vi "Status Bar.vi"(0 "Status Bar":refnum<vi>, 5 "Status":string, 11 "error in (no error)":errorcluster, 13 "Operation":T1) -> (15 "error out":errorcluster)   [LabVIEW 2014, in "SLL Application.lvlib"]
uses:
  SLL Application.lvlib
  _Typedefs/Status Bar Operation.ctl
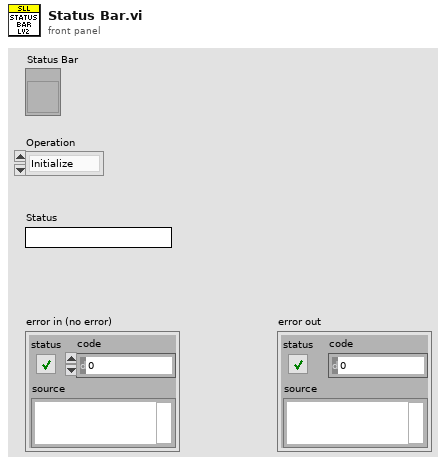
[diagram p1: front panel]
types:
  T1 = typedef "SLL Application.lvlib/Status Bar Operation.ctl" = enum16{"Initialize", "Update", "Clear", "Close"}
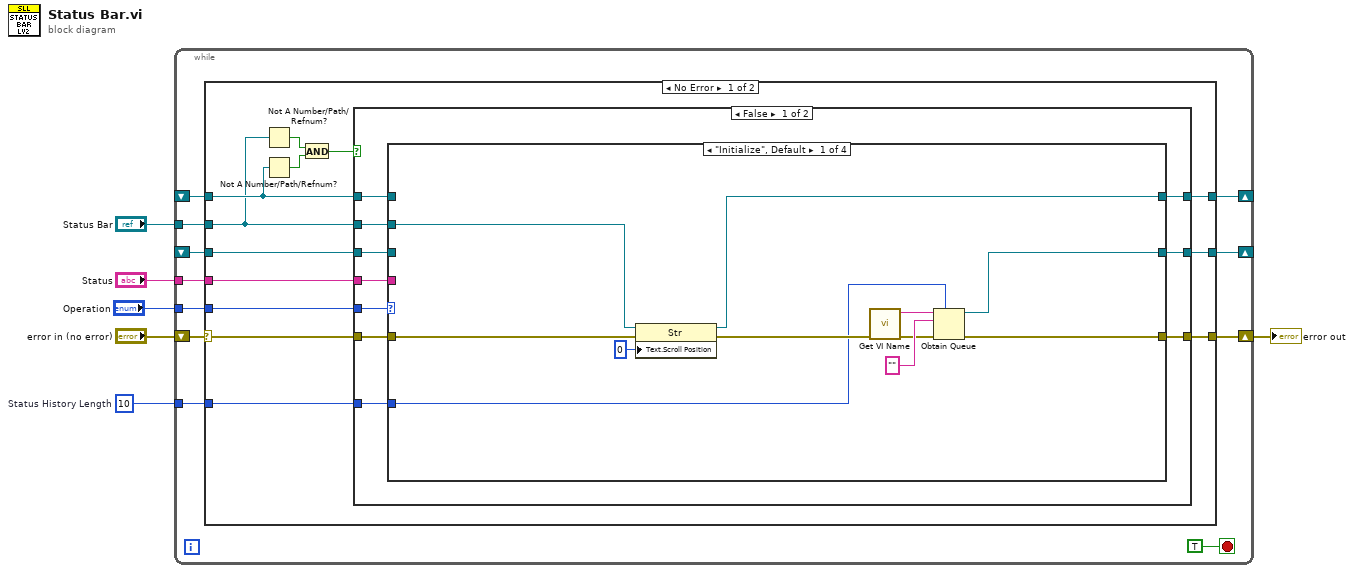
[diagram p0: block diagram]
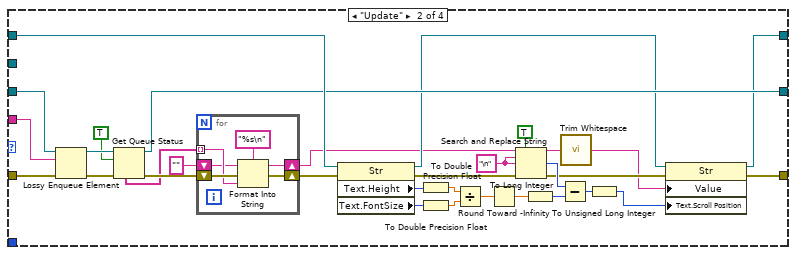
[diagram p2: hidden frame]
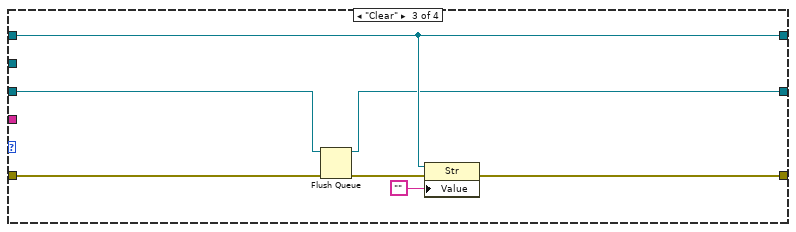
[diagram p3: hidden frame]
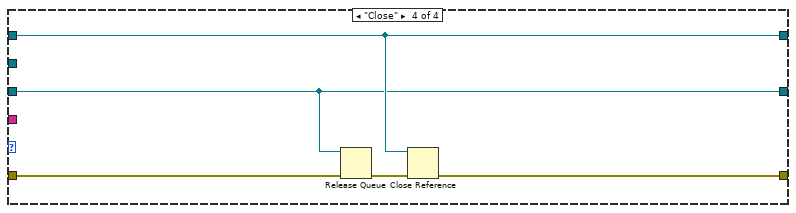
[diagram p4: hidden frame]
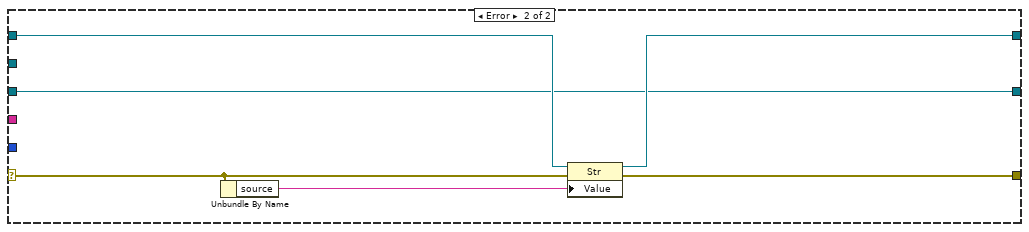
[diagram p6: hidden frame]
diagram:
  w1 = 10  # Status History Length
  n1 = while {
    shift-right: [w16] -> _
    shift-left: _ -> [w17]
    tunnel: "Operation" -> [w15]
    tunnel: "Status Bar" -> [w14]
    shift-right: [w12] -> w4
    shift-left: "error in (no error)" -> [w13]
    tunnel: "Status" -> [w10]
    shift-right: [w9] -> _
    shift-left: _ -> [w8]
    tunnel: w1 -> [w7]
    stop <- TRUE stop-if-true
    n2 = case shown="No Error" w13 {
      selector: w13 -> [w28 w107]
      tunnel: w17 -> [w20 w109]
      tunnel: [w30 w108] -> w16
      tunnel: w15 -> [w29 _]
      tunnel: w14 -> [w19 _]
      tunnel: [w27 w110] -> w12
      tunnel: w10 -> [w26 _]
      tunnel: [w25 w105] -> w9
      tunnel: w8 -> [w24 w105]
      tunnel: w7 -> [w18 _]
      frame No Error {
        n3 = Not A Number/Path/Refnum?(number/path/refnum=w19) -> (NaN/Path/Refnum?=w23:bool)
        n4 = Not A Number/Path/Refnum?(number/path/refnum=w20) -> (NaN/Path/Refnum?=w22:bool)
        n5 = And(x=w23, y=w22) -> (x .and. y?=w21:bool)
        n6 = case shown="False" w21 {
          tunnel: w20 -> [w40 w104]
          tunnel: [w39 w104] -> w30
          tunnel: w29 -> [w38 _]
          tunnel: w19 -> [w37 _]
          tunnel: w28 -> [w36 w102]
          tunnel: [w35 w102] -> w27
          tunnel: w26 -> [w34 _]
          tunnel: [w33 w103] -> w25
          tunnel: w24 -> [w32 w103]
          tunnel: w18 -> [w31 _]
          frame False {
            n7 = case shown="\"Initialize\", Default" w38 {
              tunnel: w40 -> [_ w80 w94 w100]
              tunnel: [w45 w57 w94 w100] -> w39
              tunnel: w37 -> [w46 _ _ _]
              tunnel: w36 -> [w48 w82 w95 w99]
              tunnel: [w51 w83 w96 w101] -> w35
              tunnel: w34 -> [_ w81 _ _]
              tunnel: [w49 w78 w92 w97] -> w33
              tunnel: w32 -> [_ w79 w93 w97]
              tunnel: w31 -> [w41 _ _ _]
              frame "Initialize", Default {
                n8 = property class="Str"(reference=w46, error in=w48, "Text.Scroll Position"=u32 0) -> (reference out=w45:refnum<vi>, error out=w47:errorcluster)
                n9 = call "Get VI Name.vi"("error in (no error)"=w47) -> ("error out"=w43:errorcluster, "VI Name"=w42:string)  [unwired: 9 in]
                n10 = Obtain Queue(max queue size (-1, unlimited)=w41, name (unnamed)=w42, element data type="" ("Status"), error in (no error)=w43) -> (queue out=w49:refnum<queue>, error out=w51:errorcluster)  [unwired: 1 in, 1 out]
              }
              frame "Update" {
                w63 = "\n" ("String")
                n11 = Lossy Enqueue Element(queue=w79, element=w81, error in (no error)=w82) -> (queue out=w75:refnum<queue>, error out=w77:errorcluster)  [unwired: 2 out]
                n12 = Get Queue Status(queue=w75, return elements? (F)=TRUE, error in (no error)=w77) -> (queue out=w78:refnum<queue>, error out=w76:errorcluster, elements=w73:string[])  [unwired: 5 out]
                n13 = for {
                  shift-right: [w89] -> w71
                  shift-left: w76 -> [w86]
                  tunnel: w73 -> [w85] mode=indexing
                  shift-right: [w87] -> w53
                  shift-left: "" ("Status") -> [w84]
                  n14 = Format Into String(format string="%s\n" ("Status"), initial string=w84, error in=w86, w85) -> (resulting string=w87:string, error out=w89:errorcluster)
                }
                n15 = property class="Str"(reference=w80, error in=w71) -> (reference out=w68:refnum<vi>, error out=w62:errorcluster, "Text.Height"=w70:u32, "Text.FontSize"=w69:u32)
                n16 = To Double Precision Float(number=w70) -> (double precision float=w59:dbl)
                n17 = To Double Precision Float(number=w69) -> (double precision float=w60:dbl)
                n18 = Divide(x=w59, y=w60) -> (x/y=w54:dbl)
                n19 = Round Toward -Infinity(1:w54) -> (0:w52:dbl)
                n20 = Search and Replace String(replace all?=TRUE ("replace all? (F)"), input string=w53, search string=w63, replace string=w63, error in=w62) -> (result string=w56:string, number of replacements=w65:i32, error out=w61:errorcluster)  [unwired: 3 in, 1 out]
                n21 = To Long Integer(number=w52) -> (32bit integer=w66:i32)
                n22 = Subtract(x=w65, y=w66) -> (x-y=w67:i32)
                n23 = call <vilib>:"Trim Whitespace.vi"("string"=w56) -> ("trimmed string"=w55:string)  [unwired: 1 in]
                n24 = To Unsigned Long Integer(number=w67) -> (unsigned 32bit integer=w58:u32)
                n25 = property class="Str"(reference=w68, error in=w61, "Value"=w55, "Text.Scroll Position"=w58) -> (reference out=w57:refnum<vi>, error out=w83:errorcluster)
              }
              frame "Clear" {
                n26 = Flush Queue(queue=w93, error in (no error)=w95) -> (queue out=w92:refnum<queue>, error out=w90:errorcluster)  [unwired: 1 out]
                n27 = property class="Str"(reference=w94, error in=w90, "Value"="") -> (error out=w96:errorcluster)  [unwired: 1 out]
              }
              frame "Close" {
                n28 = Release Queue(queue=w97, error in (no error)=w99) -> (error out=w98:errorcluster)  [unwired: 1 in, 2 out]
                n29 = Close Reference(reference=w100, error in (no error)=w98) -> (error out=w101:errorcluster)
              }
            }
          }
          frame True {
          }
        }
      }
      frame Error {
        n30 = Unbundle By Name(w107) -> ("source"=w106:string)
        n31 = property class="Str"(reference=w109, error in=w107, "Value"=w106) -> (reference out=w108:refnum<vi>, error out=w110:errorcluster)
      }
    }
  }
  "error out" <- w4
